vi "subIsInstanceVI.vi"(11 "delimited name":string) -> (3 "found?":bool)   [LabVIEW 2020, in "DependencyInspection.lvlib" / "CDependencyInspection.lvclass"]
uses:
  CDependencyInspection.lvclass
  CommonHelpers/CommonHelpers.lvlib
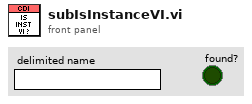
[diagram p1: front panel]
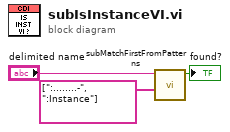
[diagram p0: block diagram]
diagram:
  n1 = call "subMatchFirstFromPatterns.vi"("patterns"=string[] [":........-", ":Instance"], "string in"="delimited name") -> ("found?"=→"found?":bool)  [unwired: 7 in, 2 out]
